vi "MTS_GetFileFromWS.vi"(10 "Tree Label":string, 11 ".pt3 File Name":path) -> (2 "File Header":T1, 3 "File Found":bool)   [LabVIEW 8.6]
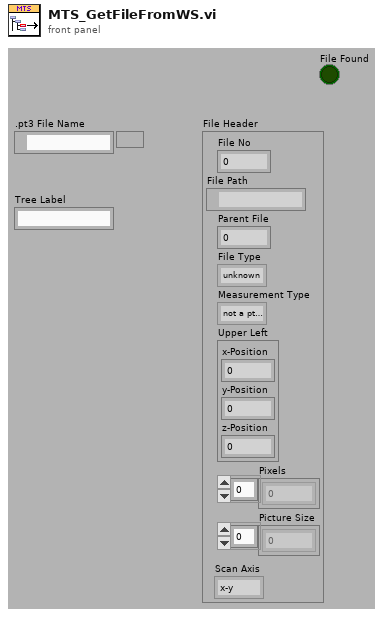
[diagram p1: front panel]
types:
  T1 = cluster{"File No":i32, "File Path":path, "Parent File":i32, "File Type":enum16{"unknown", "pt3 File", "png Image", "bmp Image"}, "Measurement Type":enum16{"not a pt3 File", "Image File", "Point Measurement", "Auto Point"}, "Upper Left":cluster{"x-Position":dbl, "y-Position":dbl, "z-Position":dbl}, "Pixels":i32[], "Picture Size":dbl[], "Scan Axis":enum32{"x-y", "x-z", "y-z"}}
  T2 = enum16{"Get (Default)", "Set Workspace", "Append File", "Change Comment"}
  T3 = cluster{"File No":i32, "File Path":path, "Parent File":i32, "File Type":enum16{"unknown", "pt3 File", "png Image", "bmp Image"}, "Measurement Type":enum16{"not a pt3 File", "Image File", "Point Measurement", "Auto Point"}, "Upper Left":cluster{"x-Position":dbl, "y-Position":dbl, "z-Position":dbl}, "Pixels":i32[], "Picture Size":dbl[], "Scan Axis":enum32{"x-y", "x-z", "y-z"}}[]
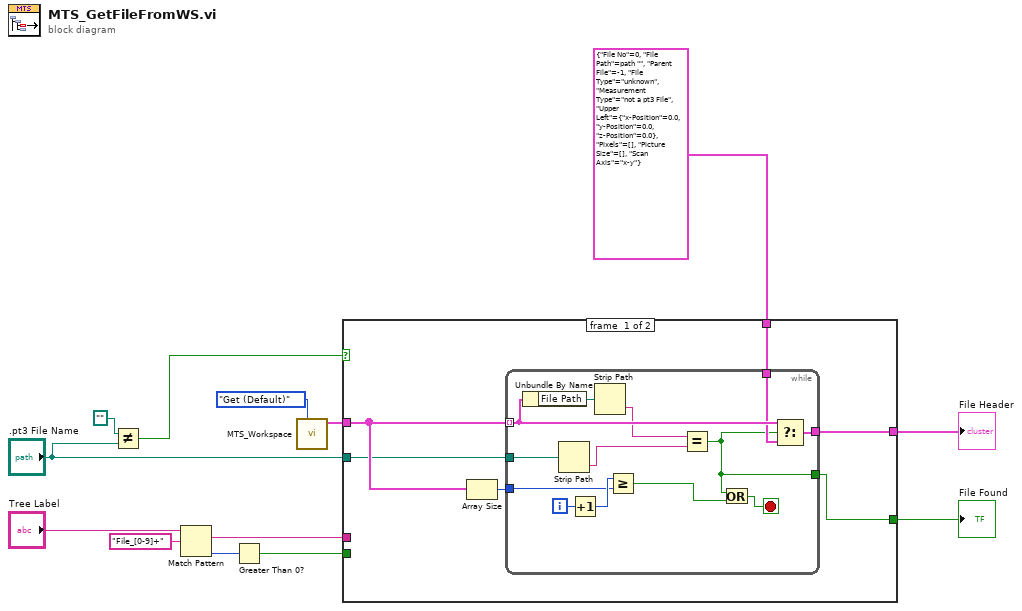
[diagram p0: block diagram]
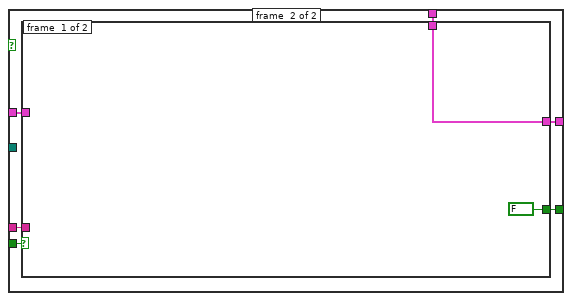
[diagram p2: hidden frame]
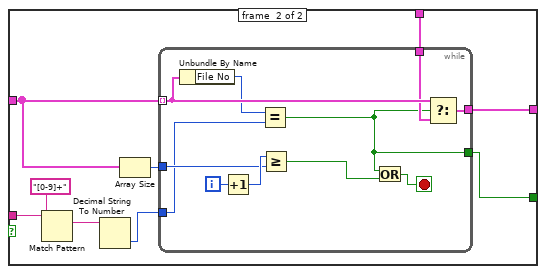
[diagram p3: hidden frame]
diagram:
  n1 = Not Equal?(x=path "", y=".pt3 File Name") -> (x != y?=w6:bool)
  n2 = Match Pattern(string="Tree Label", regular expression="File_[0-9]+") -> (match substring=w1:string, offset past match=w3:i32)  [unwired: 1 in, 2 out]
  n3 = Greater Than 0?(x=w3) -> (x > 0?=w2:bool)
  n4 = call "MTS_Workspace.vi"("Operation"=T2."Get (Default)") -> ("Files in Workspace"=w12:T3)  [unwired: 7 in, 3 out]
  n5 = case shown="False" w6 {
    tunnel: [w19 w38] -> w13
    tunnel: w12 -> [w17 w37]
    tunnel: T1 {"File No"=0, "File Path"=path "", "Parent File"=-1, "File Type"=enum."unknown", "Measurement Type"=enum."not a pt3 File", "Upper Left"={"x-Position"=0.0, "y-Position"=0.0, "z-Position"=0.0}, "Pixels"=[], "Picture Size"=[], "Scan Axis"=enum."x-y"} ("f") -> [w16 w36]
    tunnel: [w15 w35] -> w9
    tunnel: ".pt3 File Name" -> [w14 _]
    tunnel: w2 -> [_ w34]
    tunnel: w1 -> [_ w33]
    frame #0 {
      n6 = Array Size(array=w17) -> (size(s)=w18:i32)
      n7 = while {
        tunnel: w17 -> [w27] mode=indexing
        tunnel: w14 -> [w24]
        tunnel: w18 -> [w30]
        tunnel: [w26] -> w19
        tunnel: w16 -> [w21]
        tunnel: [w20] -> w15
        i -> [w32]
        stop <- w28 stop-if-true
        n8 = Unbundle By Name(w27) -> ("File Path"=w25:path)
        n9 = Strip Path(path=w24) -> (name=w22:string)  [unwired: 1 out]
        n10 = Increment(x=w32) -> (x+1=w31:i32)
        n11 = Strip Path(path=w25) -> (name=w23:string)  [unwired: 1 out]
        n12 = Greater Or Equal?(x=w31, y=w30) -> (x >= y?=w29:bool)
        n13 = Equal?(x=w23, y=w22) -> (x = y?=w20:bool)
        n14 = Or(x=w20, y=w29) -> (x .or. y?=w28:bool)
        n15 = Select(t=w27, s=w20, f=w21) -> (s? t:f=w26:T1)
      }
    }
    frame #1 {
      n16 = case shown="True" w34 {
        tunnel: [w40 w49] -> w38
        tunnel: w37 -> [_ w47]
        tunnel: w36 -> [w40 w46]
        tunnel: [FALSE w45] -> w35
        tunnel: w33 -> [_ w44]
        frame #0 {
        }
        frame #1 {
          n17 = Match Pattern(string=w44, regular expression="[0-9]+") -> (match substring=w42:string)  [unwired: 1 in, 3 out]
          n18 = Decimal String To Number(string=w42) -> (number=w41:i32)  [unwired: 2 in, 1 out]
          n19 = Array Size(array=w47) -> (size(s)=w48:i32)
          n20 = while {
            tunnel: w47 -> [w55] mode=indexing
            tunnel: w48 -> [w58]
            tunnel: [w54] -> w49
            tunnel: w46 -> [w53]
            tunnel: [w50] -> w45
            tunnel: w41 -> [w51]
            i -> [w60]
            stop <- w56 stop-if-true
            n21 = Unbundle By Name(w55) -> ("File No"=w52:i32)
            n22 = Increment(x=w60) -> (x+1=w59:i32)
            n23 = Equal?(x=w52, y=w51) -> (x = y?=w50:bool)
            n24 = Greater Or Equal?(x=w59, y=w58) -> (x >= y?=w57:bool)
            n25 = Or(x=w50, y=w57) -> (x .or. y?=w56:bool)
            n26 = Select(t=w55, s=w50, f=w53) -> (s? t:f=w54:T1)
          }
        }
      }
    }
  }
  "File Header" <- w13
  "File Found" <- w9
